vi "LifeTimeImagePoint.vi"(0 "Boolean in":refnum<vi>, 3 "String":string, 4 "reference 6":refnum<vi>, 5 "String 2":string, 6 "reference 7":refnum<vi>, 7 "error in (no error)":errorcluster, 8 "reference 4":refnum<vi>, 10 "reference 3":refnum<vi>, 11 "reference 9":refnum<vi>, 12 "reference in":refnum<vi>, 13 "DigNum Refnum":refnum<vi>, 14 "Numeric in":i32, 15 "Str Refnum":refnum<vi>, 16 "X Stepsize":dbl, 18 "Array in":i32[][](array[numeric]), 19 "Point Measurement":refnum<vi>) -> (20 "Array out":i32[][](array[numeric]), 21 "CCD Chip Size":i32, 22 "X Start":dbl, 23 "Numeric out":dbl, 27 "error out":errorcluster)   [LabVIEW 2011]
uses:
  Camera/vi/CamDef.vi
  Camera/lib/System Files/user.lib/atmcd32d.llb/Error Code Enum typedef.ctl
  Camera/vi/ccdChipPixels.vi
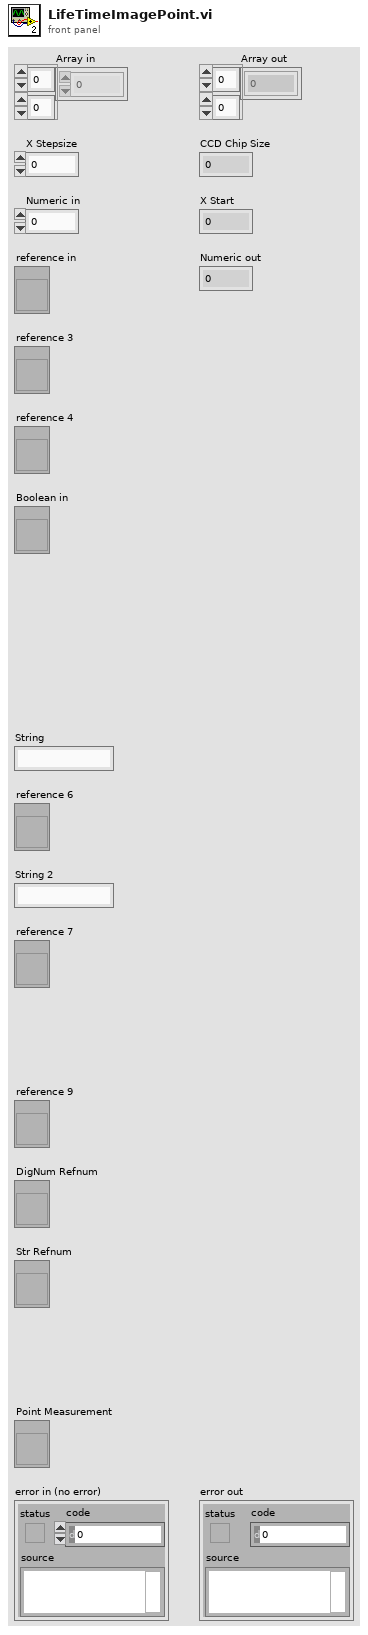
[diagram p1: front panel]
types:
  T1 = enum16{"No Measurement", "Aquire Image", "Point Measurement", "Multi Measurement", "Save Color Image"}
  T2 = enum16{"No Measurement", "Aquire Image", "Point Measurement", "Multi Measurement", "Save Color Image", "Find Single Mol.", "Auto Measurement Control", "Auto Point", "Aquire Line Scan", "Grid Measurement", "Trapping", "Move Scanner"}
  T3 = typedef "Error Code Enum typedef.ctl" = enum32{"N/A (0)", "DRV_ERROR_CODES", "DRV_SUCCESS", "DRV_VXDNOTINSTALLED", "DRV_ERROR_SCAN", "DRV_ERROR_CHECK_SUM", "DRV_ERROR_FILELOAD", "DRV_UNKNOWN_FUNC", "DRV_ERROR_VXD_INIT", "DRV_ERROR_ADDRESS", "DRV_ERROR_PAGELOCK", "DRV_ERROR_PAGEUNLOCK", "DRV_ERROR_BOARDTEST", "DRV_ERROR_ACK", "DRV_ERROR_UP_FIFO", "DRV_ERROR_PATTERN", "N/A (16)", "DRV_ACQUISITION_ERRORS", "DRV_ACQ_BUFFER", "DRV_ACQ_DOWNFIFO_FULL", "DRV_PROC_UNKONWN_INSTRUCTION", "DRV_ILLEGAL_OP_CODE", "DRV_KINETIC_TIME_NOT_MET", "DRV_ACCUM_TIME_NOT_MET", "DRV_NO_NEW_DATA", "N/A (25)", "DRV_SPOOLERROR", "N/A (27)", "N/A (28)", "N/A (29)", "N/A (30)", "N/A (31)", "N/A (32)", "DRV_TEMPERATURE_CODES", "DRV_TEMPERATURE_OFF", "DRV_TEMPERATURE_NOT_STABILIZED", "DRV_TEMPERATURE_STABILIZED", "DRV_TEMPERATURE_NOT_REACHED", "DRV_TEMPERATURE_OUT_RANGE", "DRV_TEMPERATURE_NOT_SUPPORTED", "DRV_TEMPERATURE_DRIFT", "N/A (41)", "N/A (42)", "N/A (43)", "N/A (44)", "N/A (45)", "N/A (46)", "N/A (47)", "N/A (48)", "DRV_GENERAL_ERRORS", "DRV_INVALID_AUX", "DRV_COF_NOTLOADED", "DRV_FPGAPROG", "DRV_FLEXERROR", "DRV_GPIBERROR", "N/A (55)", "N/A (56)", "N/A (57)", "N/A (58)", "N/A (59)", "N/A (60)", "N/A (61)", "N/A (62)", "N/A (63)", "DRV_DATATYPE", "DRV_DRIVER_ERRORS", "DRV_P1INVALID", "DRV_P2INVALID", "DRV_P3INVALID", "DRV_P4INVALID", "DRV_INIERROR", "DRV_COFERROR", "DRV_ACQUIRING", "DRV_IDLE", "DRV_TEMPCYCLE", "DRV_NOT_INITIALIZED", "DRV_P5INVALID", "DRV_P6INVALID", "DRV_INVALID_MODE", "DRV_INVALID_FILTER", "DRV_I2CERRORS", "DRV_I2CDEVNOTFOUND", "DRV_I2CTIMEOUT", "DRV_P7INVALID", "N/A (84)", "N/A (85)", "N/A (86)", "N/A (87)", "N/A (88)", "N/A (89)", "DRV_IOCERROR", "DRV_VRMVERSIONERROR"}
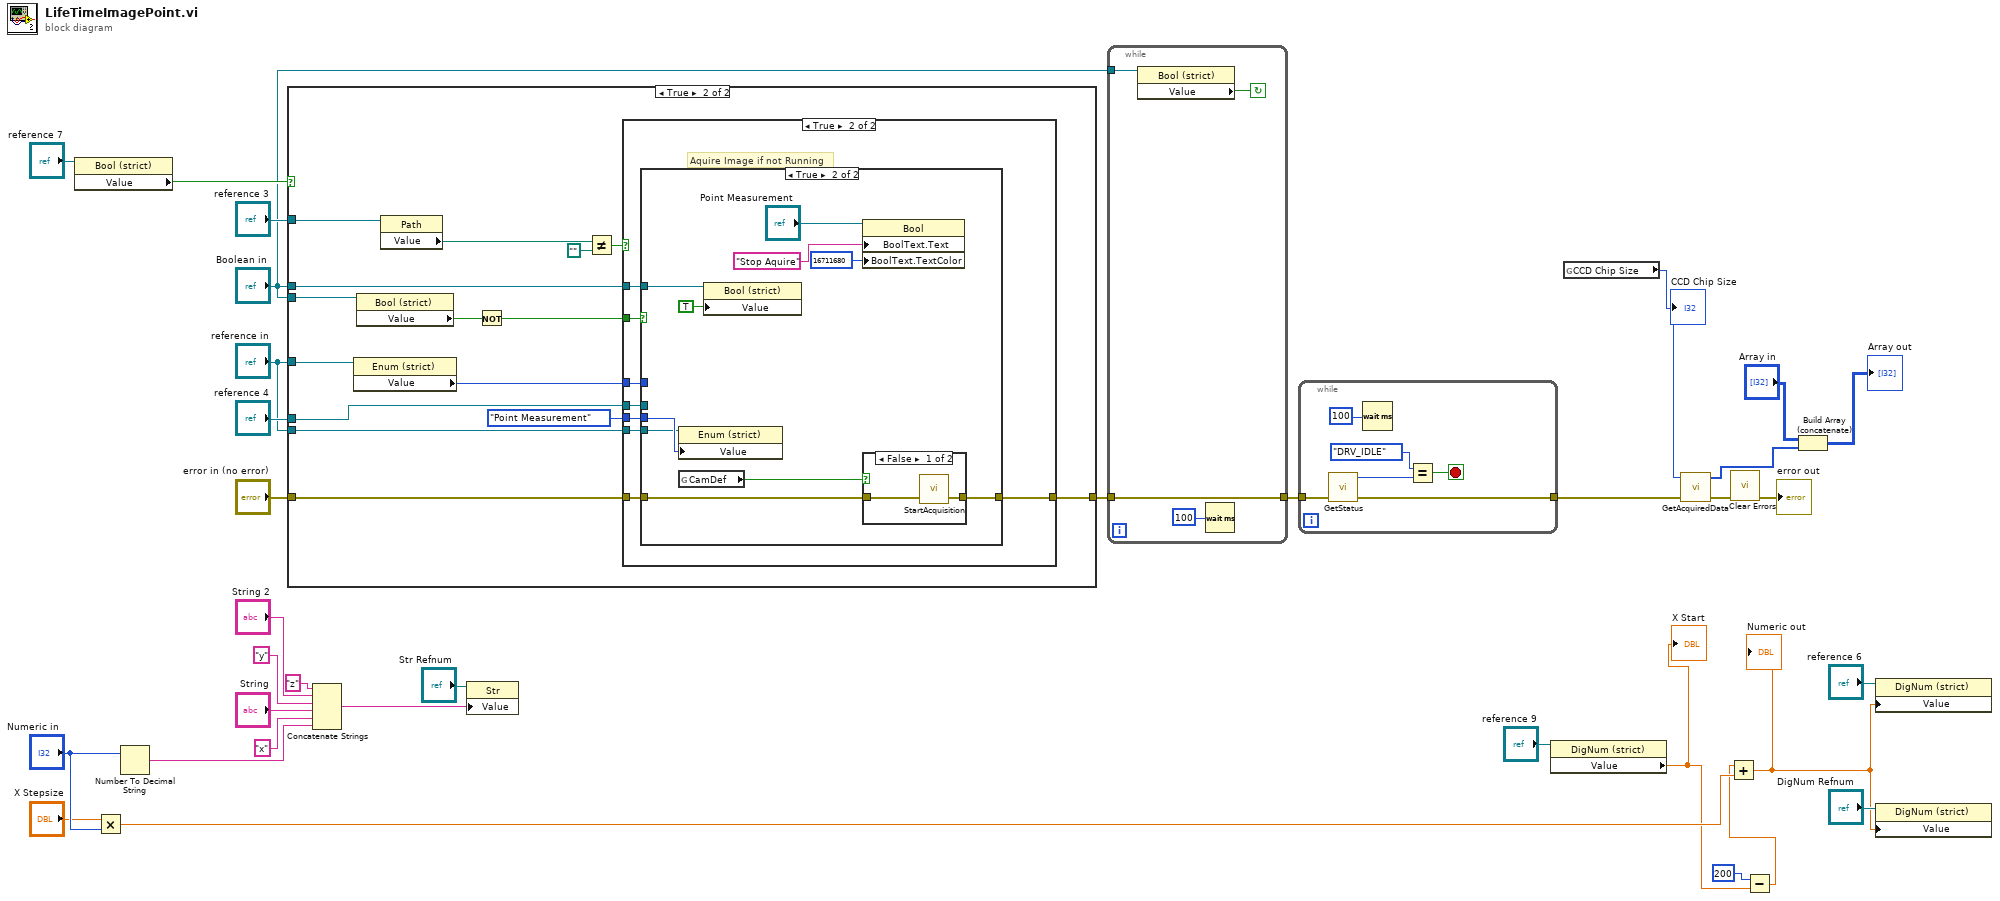
[diagram p0: block diagram]
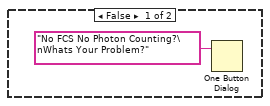
[diagram p2: hidden frame]
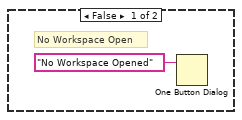
[diagram p3: hidden frame]
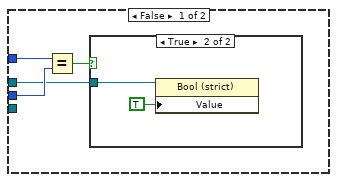
[diagram p4: hidden frame]
diagram:
  n1 = property class="Bool (strict)"(reference="reference 7") -> ("Value"=w24:bool)  [unwired: 1 in, 2 out]
  n2 = Multiply(x="X Stepsize", y="Numeric in") -> (x*y=w25:dbl)
  n3 = Number To Decimal String(number="Numeric in") -> (decimal integer string=w23:string)  [unwired: 1 in]
  n4 = case shown="True" w24 {
    tunnel: [_ w44] -> w15
    tunnel: "error in (no error)" -> [_ w43]
    tunnel: "Boolean in" -> [_ w41]
    tunnel: "reference in" -> [_ w40]
    tunnel: "reference 3" -> [_ w39]
    tunnel: "reference 4" -> [_ w38]
    tunnel: "reference in" -> [_ w37]
    tunnel: "Boolean in" -> [_ w36]
    frame False {
      n5 = One Button Dialog(message="No FCS No Photon Counting?\nWhats Your Problem?") -> ()  [unwired: 1 in, 1 out]
    }
    frame True {
      n6 = property class="Enum (strict)"(reference=w40) -> ("Value"=w49:T2)  [unwired: 1 in, 2 out]
      n7 = property class="Bool (strict)"(reference=w41) -> ("Value"=w50:bool)  [unwired: 1 in, 2 out]
      n8 = property class="Path"(reference=w39) -> ("Value"=w42:path)  [unwired: 1 in, 2 out]
      n9 = Not(x=w50) -> (.not. x?=w45:bool)
      n10 = Not Equal?(x=w42, y=path "") -> (x != y?=w46:bool)
      n11 = case shown="True" w46 {
        tunnel: w45 -> [_ w59]
        tunnel: T1."Point Measurement" ("Do Measurement") -> [_ w58]
        tunnel: w49 -> [_ w57]
        tunnel: [_ w56] -> w44
        tunnel: w43 -> [_ w55]
        tunnel: w38 -> [_ w54]
        tunnel: w37 -> [_ w53]
        tunnel: w36 -> [_ w52]
        frame False {
          # "No Workspace Open"
          n12 = One Button Dialog(message="No Workspace Opened") -> ()  [unwired: 1 in, 1 out]
        }
        frame True {
          # "Aquire Image if not Running"
          n13 = case shown="True" w59 {
            tunnel: w58 -> [w62 w73]
            tunnel: w57 -> [w63 _]
            tunnel: [_ w70] -> w56
            tunnel: w55 -> [_ w69]
            tunnel: w54 -> [w60 _]
            tunnel: w53 -> [_ w67]
            tunnel: w52 -> [_ w66]
            frame False {
              n14 = Equal?(x=w63, y=w62) -> (x = y?=w61:bool)
              n15 = case shown="True" w61 {
                tunnel: w60 -> [_ w64]
                frame False {
                }
                frame True {
                  n16 = property class="Bool (strict)"(reference=w64, "Value"=TRUE ("Stop Measurement")) -> ()  [unwired: 1 in, 2 out]
                }
              }
            }
            frame True {
              n17 = property class="Enum (strict)"(reference=w67, "Value"=w73) -> ()  [unwired: 1 in, 2 out]
              n18 = global read "CamDef.vi" "CamDef"() -> (w68:bool)
              n19 = property class="Bool (strict)"(reference=w66, "Value"=TRUE ("Measurement Running")) -> ()  [unwired: 1 in, 2 out]
              n20 = property on="Property Node" class="Bool"(reference="Point Measurement", "BoolText.Text"="Stop Aquire" ("Caption.Text"), "BoolText.TextColor"=u32 16711680 ("Boolean Text.Colors:FG Color")) -> ()  [unwired: 1 in, 2 out]
              n21 = case shown="False" w68 {
                tunnel: [w76 w78] -> w70
                tunnel: w69 -> [w77 w78]
                frame False {
                  n22 = call "StartAcquisition.vi"("error in (no error)"=w77) -> ("error out"=w76:errorcluster)  [unwired: 1 in, 1 out]
                }
                frame True {
                }
              }
            }
          }
        }
      }
    }
  }
  n23 = Concatenate Strings("z" ("string"), "String 2", "y" ("string"), "String", "x" ("string"), w23) -> (w34:string)
  n24 = property on="Property Node" class="Str"(reference="Str Refnum", "Value"=w34) -> ()  [unwired: 1 in, 2 out]
  n25 = while {
    tunnel: w15 -> [w79]
    tunnel: [w79] -> w28
    tunnel: "Boolean in" -> [w80]
    stop <- w82 continue-if-true
    n26 = property class="Bool (strict)"(reference=w80) -> ("Value"=w82:bool)  [unwired: 1 in, 2 out]
    n27 = Wait (ms)(milliseconds to wait=u32 100) -> ()  [unwired: 1 out]
  }
  n28 = while {
    tunnel: w28 -> [w83]
    tunnel: [w86] -> w27
    stop <- w85 stop-if-true
    n29 = call "GetStatus.vi"("error in (no error)"=w83) -> ("error out"=w86:errorcluster, "status"=w87:T3)  [unwired: 2 in, 1 out]
    n30 = Wait (ms)(milliseconds to wait=u32 100) -> ()  [unwired: 1 out]
    n31 = Equal?(x=Error_Code_Enum_typedef."DRV_IDLE" ("status"), y=w87) -> (x = y?=w85:bool)
  }
  n32 = property class="DigNum (strict)"(reference="reference 9") -> ("Value"=w3:dbl)  [unwired: 1 in, 2 out]
  "X Start" <- w3
  n33 = global read "ccdChipPixels.vi" "CCD Chip Size"() -> (w33:i32)
  "CCD Chip Size" <- w33
  n34 = call "GetAcquiredData.vi"("error in (no error)"=w27, "size"=w33) -> ("error out"=w29:errorcluster, "array"=w30:i32[])  [unwired: 1 in, 1 out]
  n35 = call <vilib>:"Clear Errors.vi"("error in (no error)"=w29) -> ("error out"=→"error out":errorcluster)  [unwired: 6 in]
  n36 = Subtract(x=200, y=w3) -> (x-y=w2:dbl)
  n37 = Add(x=w2, y=w25) -> (x+y=w1:dbl)
  "Numeric out" <- w1
  n38 = Build Array (concatenate)("Array in", w30) -> (→"Array out":i32[][])
  n39 = property class="DigNum (strict)"(reference="reference 6", "Value"=w1) -> ()  [unwired: 1 in, 2 out]
  n40 = property on="Property Node" class="DigNum (strict)"(reference="DigNum Refnum", "Value"=w1) -> ()  [unwired: 1 in, 2 out]
